vi "lv_UART.vi"() -> ()   [LabVIEW 2018]
uses:
  <vilib>/Instr/_visa.llb/VISA Open Access Mode.ctl
  <vilib>/Instr/_visa.llb/Select Event Type.ctl
  <vilib>/Instr/_visa.llb/VISA Event Mechanism.ctl
  <vilib>/Instr/_visa.llb/VISA Configure Serial Port (Instr).vi
panel:
  in  "VISA":refnum<visa-resource-name>="COM7"
  in  "stop":bool
  in  "Send":bool
  out "收到的数据":string
  in  "Senddata":string
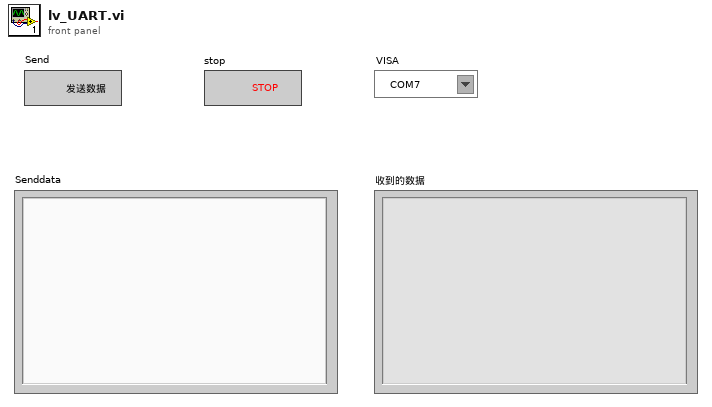
[diagram p1: front panel]
types:
  T1 = typedef "VISA Event Mechanism.ctl" = u16
  T2 = typedef "Select Event Type.ctl" = u32
  T3 = typedef "VISA Open Access Mode.ctl" = u32
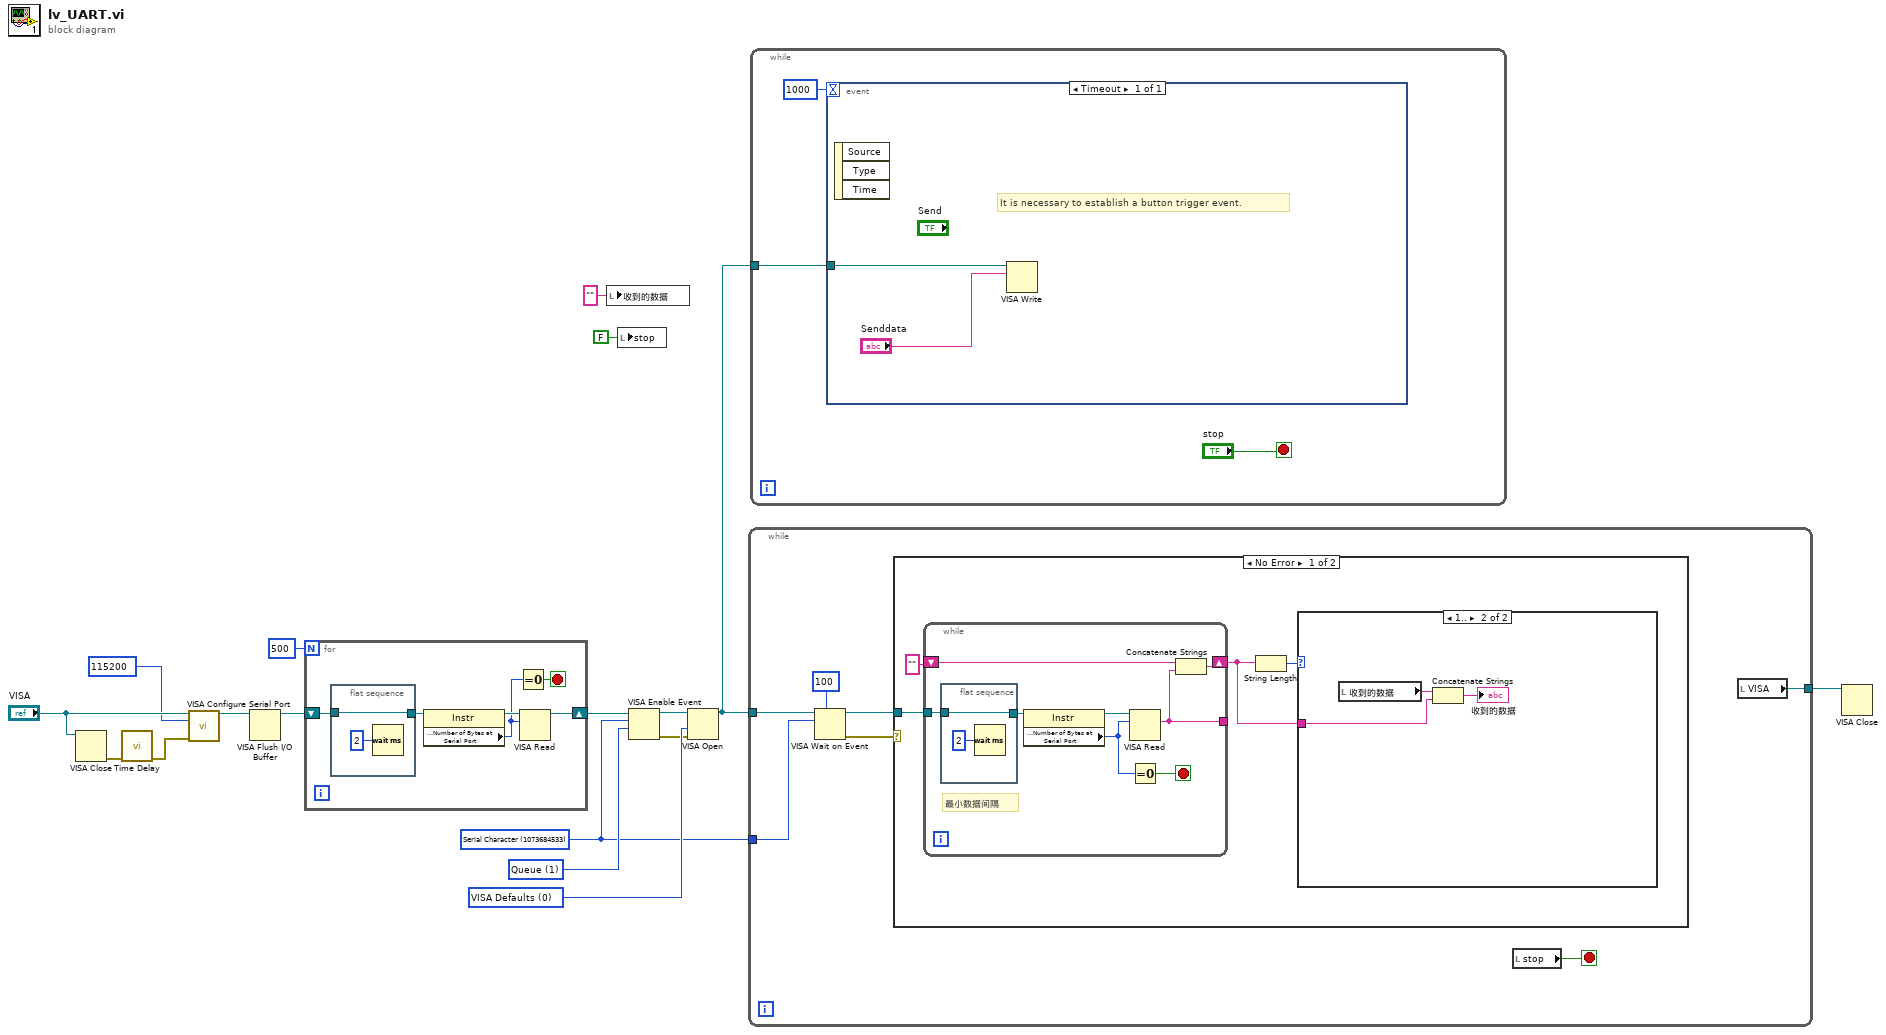
[diagram p0: block diagram]
diagram:
  w9 = T1 1 items=["Queue"=1] ("Mechanism Type")
  w7 = T2 1073684533 items=["Service Request"=1073684491, "Trigger"=3221168138, "Clear"=1073684493, "VXI Signal"=1073684512, "VXI/VME Interrupt"=3221168161, "VXI/VME Sysfail"=1073684509, "VXI/VME Sysreset"=1073684510, "GPIB CIC"=1073684498, "GPIB Talk"=1073684499, "GPIB Listen"=1073684500, "PXI Interrupt"=1073684514, "Serial Break"=1073684515, "Serial TermChar"=1073684516, "Serial CTS"=1073684521, "Serial DSR"=1073684522, "Serial DCD"=1073684524, "Serial RI"=1073684526, "Serial Character"=1073684533, "USB Interrupt"=1073684535, "All Enabled"=1073709055] ("Event Type")
  w14 = T3 0 items=["VISA Defaults"=0, "Exclusive Lock"=1, "Load Configured Settings"=4] ("Access Mode")
  n1 = VISA Close(VISA resource name="VISA") -> (error out=w16:errorcluster)  [unwired: 1 in]
  n2 = call "Time Delay"("error in (no error)"=w16) -> ("error out"=w15:errorcluster)  [unwired: 10 in]
  n3 = call-poly "VISA Configure Serial Port"("VISA resource name"="VISA", "baud rate (9600)"=u32 115200 ("baud rate"), "error in (no error)"=w15) -> ("VISA resource name out"=w2:refnum<visa-resource-name>)  [unwired: 11 in, 1 out]
  n4 = VISA Flush I/O Buffer(VISA resource name=w2) -> (VISA resource name out=w1:refnum<visa-resource-name>)  [unwired: 2 in, 1 out]
  n5 = for {
    N: 500 -> [_]
    shift-right: [w20] -> w11
    shift-left: w1 -> [w22]
    stop <- w18 stop-if-true
    n6 = flat-sequence {
      tunnel: [w24] -> w21
      tunnel: w22 -> [w24]
      frame #0 {
        n7 = Wait (ms)(milliseconds to wait=u32 2) -> ()  [unwired: 1 out]
      }
    }
    n8 = property class="Instr"(reference=w21) -> (reference out=w23:refnum<visa-resource-name>, "Serial Settings:Number of Bytes at Serial Port"=w19:u32)  [unwired: 1 in, 1 out]
    n9 = Equal To 0?(x=w19) -> (x = 0?=w18:bool)
    n10 = VISA Read(VISA resource name=w23, byte count=w19) -> (VISA resource name out=w20:refnum<visa-resource-name>)  [unwired: 1 in, 3 out]
  }
  n11 = local write "收到的数据"("" ("收到的数据")) -> ()
  n12 = local write "stop"(FALSE ("stop")) -> ()
  n13 = VISA Enable Event(9:w9, 10:w7, 11:w11) -> (0:w12:errorcluster, 3:w13:refnum<visa-resource-name>)  [unwired: 1 in]
  n14 = VISA Open(access mode=w14, error in (no error)=w12, VISA resource name=w13) -> (VISA resource name=w6:refnum<visa-resource-name>)  [unwired: 2 in, 1 out]
  n15 = while {
    tunnel: w6 -> [w29]
    tunnel: w7 -> [w28]
    tunnel: [w26] -> w3
    stop <- w27 stop-if-true
    n16 = VISA Wait on Event(7:u32 100 ("timeout (0)"), 10:w28, 11:w29) -> (0:w32:errorcluster, 3:w31:refnum<visa-resource-name>)  [unwired: 2 in, 2 out]
    n17 = case shown="No Error" w32 {
      tunnel: w31 -> [w36 _]
      frame No Error {
        n18 = while {
          tunnel: w36 -> [w46]
          tunnel: [w43] -> _
          shift-right: [w42] -> w33
          shift-left: "" ("read buffer") -> [w44]
          stop <- w40 stop-if-true
          # "最小数据间隔"
          n19 = flat-sequence {
            tunnel: [w48] -> w45
            tunnel: w46 -> [w48]
            frame #0 {
              n20 = Wait (ms)(milliseconds to wait=u32 2) -> ()  [unwired: 1 out]
            }
          }
          n21 = property class="Instr"(reference=w45) -> (reference out=w47:refnum<visa-resource-name>, "Serial Settings:Number of Bytes at Serial Port"=w41:u32)  [unwired: 1 in, 1 out]
          n22 = VISA Read(VISA resource name=w47, byte count=w41) -> (read buffer=w43:string)  [unwired: 1 in, 3 out]
          n23 = Equal To 0?(x=w41) -> (x = 0?=w40:bool)
          n24 = Concatenate Strings(w44, w43) -> (w42:string)
        }
        n25 = String Length(string=w33) -> (length=w34:i32)
        n26 = case shown="1.." w34 {
          tunnel: w33 -> [_ w39]
          frame 0, Default {
          }
          frame 1.. {
            n27 = local read "收到的数据"() -> (w37:string)
            n28 = Concatenate Strings(w37, w39) -> (→"收到的数据":string)
          }
        }
      }
      frame Error {
      }
    }
    n29 = local read "stop"() -> (w27:bool)
    n30 = local read "VISA"() -> (w26:refnum<visa-resource-name>)
  }
  n31 = while {
    tunnel: w6 -> [w51]
    stop <- "stop" stop-if-true
    n32 = event shown="[0] Timeout" {
      selector: _ -> [_]
      dyn-events: _ -> [_]
      timeout: 1000 -> [_]
      tunnel: w51 -> [w54]
      event Timeout {
        # "It is necessary to establish a button trigger event."
        n33 = event-data() -> ()  [unwired: 1 in, 3 out]
        n34 = VISA Write(VISA resource name=w54, write buffer="Senddata") -> ()  [unwired: 1 in, 3 out]
      }
    }
  }
  n35 = VISA Close(VISA resource name=w3) -> ()  [unwired: 1 in, 1 out]
